vi "Action.vi"(8 "error in (no error)":errorcluster, 10 "Actor in":refnum<class "Tamagotchi Basic Actor.lvclass">, 11 "Borken Arrow Message in":refnum<class "Broken Arrow Message.lvclass">) -> (0 "error out":errorcluster, 2 "Actor out":refnum<class "Tamagotchi Basic Actor.lvclass">, 3 "Borken Arrow Message out":refnum<class "Broken Arrow Message.lvclass">)   [LabVIEW 2026, in "Broken Arrow Message.lvclass"]
uses:
  Broken Arrow Message.lvclass
  Tamagotchi Basic Actor/Tamagotchi Basic Actor.lvclass
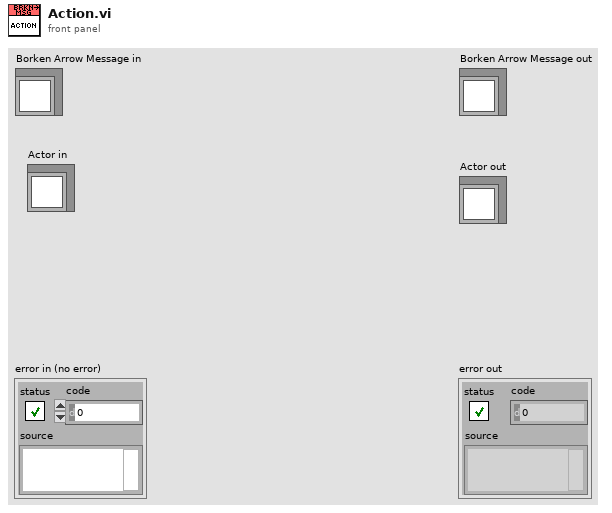
[diagram p1: front panel]
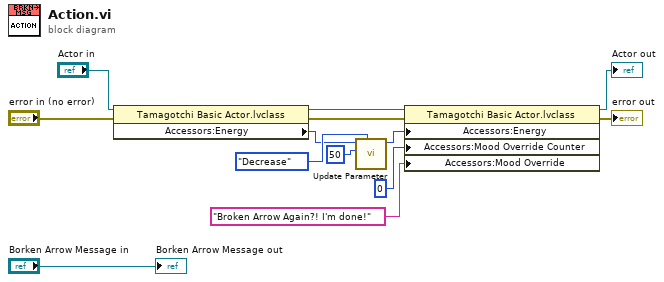
[diagram p0: block diagram]
diagram:
  n1 = property class="Tamagotchi Basic Actor.lvclass"(reference="Actor in", error in="error in (no error)") -> (reference out=w11:refnum<class "Tamagotchi Basic Actor.lvclass">, error out=w8:errorcluster, "Accessors:Energy"=w4:i16)
  n2 = call "Update Parameter.vi"("Action"=enum16{"Increase", "Decrease"}."Decrease", "Modifier"=i16 50 ("y"), "Parameter"=w4) -> ("New Value"=w3:i16)  [unwired: 8 in]
  n3 = property class="Tamagotchi Basic Actor.lvclass"(reference=w11, error in=w8, "Accessors:Energy"=w3, "Accessors:Mood Override Counter"=u32 0 ("Mood Override Counter"), "Accessors:Mood Override"="Broken Arrow Again?! I'm done!" ("Mood Override")) -> (reference out=→"Actor out":refnum<class "Tamagotchi Basic Actor.lvclass">, error out=→"error out":errorcluster)
  "Borken Arrow Message out" <- "Borken Arrow Message in"
